vi "CalcRotationAngles.vi"(7 "ZAxis":dbl, 9 "XAxis":dbl, 11 "YAxis":dbl) -> (4 "Angles":dbl[](array[numeric]), 6 "Speeds":dbl[](array[numeric]))   [LabVIEW 2018]
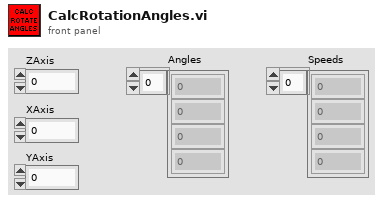
[diagram p1: front panel]
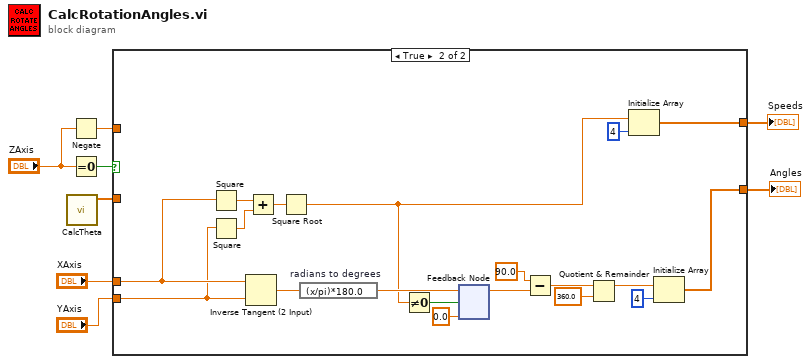
[diagram p0: block diagram]
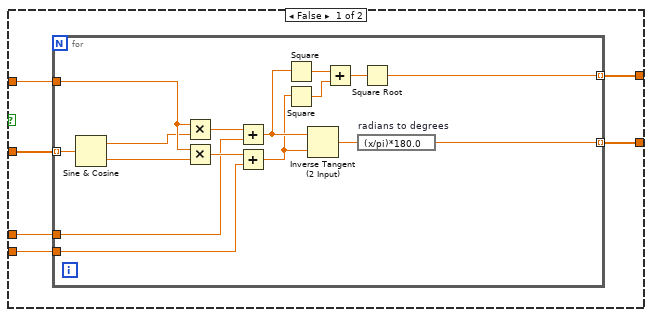
[diagram p2: hidden frame]
diagram:
  n1 = call "CalcTheta.vi"() -> ("ThetaValues"=w5:dbl[])  [unwired: 11 in]
  n2 = Negate(x="ZAxis") -> (-x=w1:dbl)
  n3 = Equal To 0?(x="ZAxis") -> (x = 0?=w7:bool)
  n4 = case shown="True" w7 {
    tunnel: [w14 w32] -> w4
    tunnel: [w13 w47] -> w8
    tunnel: w5 -> [w12 _]
    tunnel: "XAxis" -> [w11 w35]
    tunnel: "YAxis" -> [w10 w34]
    tunnel: w1 -> [w9 _]
    frame False {
      n5 = for {
        tunnel: w12 -> [w30] mode=indexing
        tunnel: w9 -> [w29]
        tunnel: w11 -> [w15]
        tunnel: w10 -> [w17]
        tunnel: [w19] -> w14 mode=indexing
        tunnel: [w20] -> w13 mode=indexing
        n6 = Sine & Cosine(0:w30) -> (1:w16:dbl, 2:w18:dbl)
        n7 = Multiply(x=w29, y=w16) -> (x*y=w27:dbl)
        n8 = Multiply(x=w29, y=w18) -> (x*y=w28:dbl)
        n9 = Add(x=w27, y=w15) -> (x+y=w25:dbl)
        n10 = Add(x=w28, y=w17) -> (x+y=w24:dbl)
        n11 = Square(x=w25) -> (x^2=w23:dbl)
        n12 = Square(x=w24) -> (x^2=w22:dbl)
        n13 = Inverse Tangent (2 Input)(1:w24, 2:w25) -> (0:w26:dbl)
        n14 = Add(x=w23, y=w22) -> (x+y=w21:dbl)
        n15 = expression code="(x/pi)*180.0" "radians to degrees"(w26) -> (w19:dbl)
        n16 = Square Root(x=w21) -> (sqrt(x)=w20:dbl)
      }
    }
    frame True {
      n17 = Square(x=w35) -> (x^2=w46:dbl)
      n18 = Square(x=w34) -> (x^2=w45:dbl)
      n19 = Inverse Tangent (2 Input)(1:w34, 2:w35) -> (0:w43:dbl)
      n20 = Add(x=w46, y=w45) -> (x+y=w44:dbl)
      n21 = Square Root(x=w44) -> (sqrt(x)=w31:dbl)
      n22 = expression code="(x/pi)*180.0" "radians to degrees"(w43) -> (w36:dbl)
      n23 = Not Equal To 0?(x=w31) -> (x != 0?=w37:bool)
      n24 = feedback #1(0.0) -> (w41:dbl)
      n25 = feedback-in #1(w36, w37) -> ()
      n26 = Subtract(x=90.0, y=w41) -> (x-y=w42:dbl)
      n27 = Quotient & Remainder(x=w42, y=360.0) -> (x-y*floor(x/y)=w33:dbl)  [unwired: 1 out]
      n28 = Initialize Array(w31, 4 ("dimension size")) -> (w47:dbl[])
      n29 = Initialize Array(w33, 4 ("dimension size")) -> (w32:dbl[])
    }
  }
  "Angles" <- w4
  "Speeds" <- w8
